vi "VecBuilder_8x1Fill.vi"(4 "R7":dbl, 5 "R0":dbl, 6 "R6":dbl, 7 "R1":dbl, 8 "R5":dbl, 9 "R4":dbl, 10 "R3":dbl, 11 "R2":dbl) -> (3 "output matrix":T1)   [LabVIEW 2019, in "Trajectory_Library.lvlib"]
doc: "Build a 8 x 1 Matrix (vector) from an array of input values.\n\nInputs:\n -- R0 -- Input value 1\n -- R1 -- Input value 2\n -- R2 -- Input value 3\n -- R3 -- Input value 4\n -- R4 -- Input value 5\n -- R5 -- Input value 6\n -- R6 -- Input value 7\n -- R7 -- Input value 8\n\nOutputs:\n -- Output Matrix -- Resulting 8 x 1 matrix (vector)"
uses:
  Trajectory_Library.lvlib
  <vilib>/Analysis/Matrix/Datatypes/RealMatrix.ctl
  <vilib>/Analysis/Matrix/NI_Matrix.lvlib
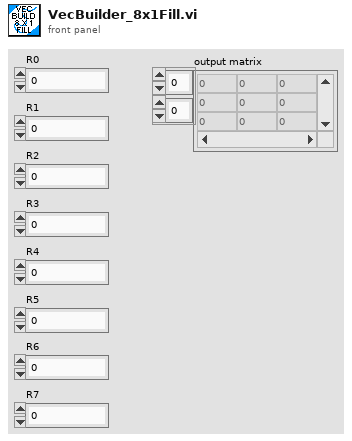
[diagram p1: front panel]
types:
  T1 = typedef "NI_Matrix.lvlib/RealMatrix.ctl" = dbl[][]
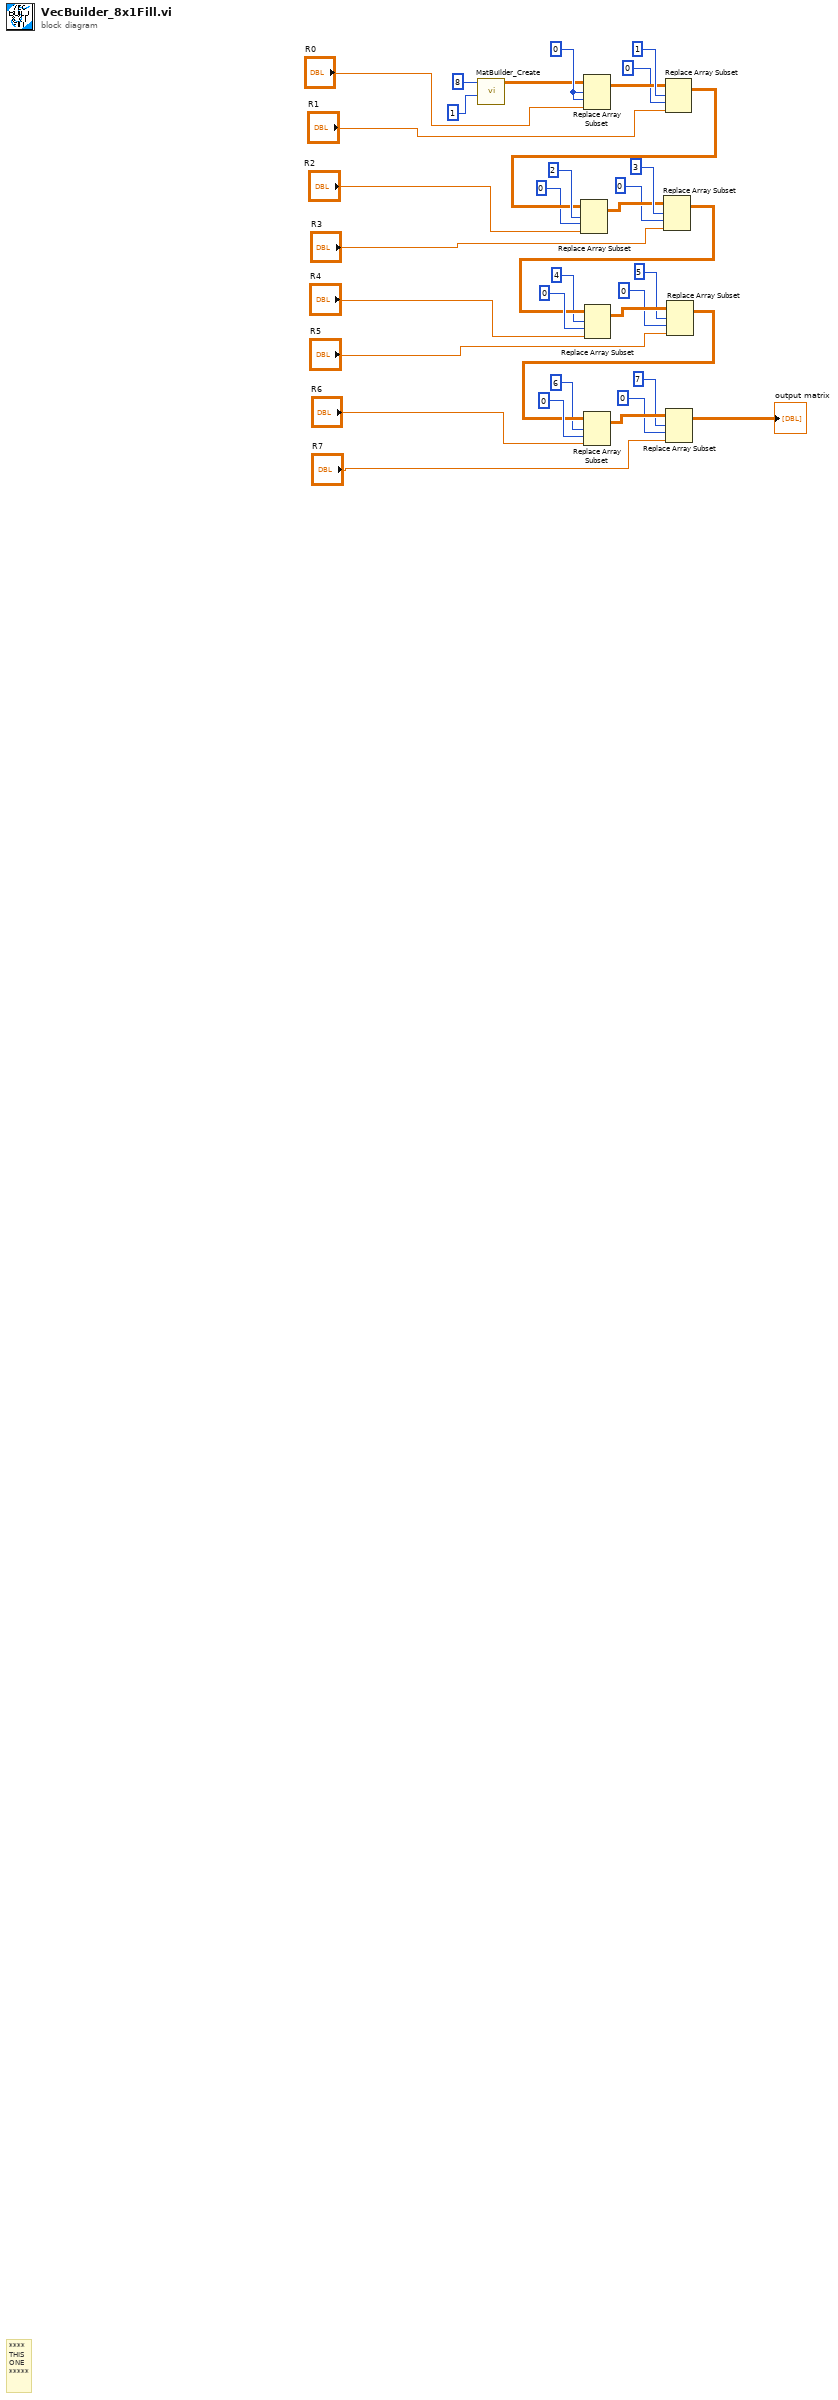
[diagram p0: block diagram]
diagram:
  w34 = 0 ("index (col)")
  # "****\nTHIS\nONE\n*****"
  n1 = call "MatBuilder_Create.vi"("Columns"=1, "Rows"=8) -> ("output matrix"=w22:T1)  [unwired: 9 in]
  n2 = Replace Array Subset(array=w22, new element="R0", index (row)=w34, index (col)=w34) -> (w32:T1)
  n3 = Replace Array Subset(array=w32, new element="R1", index (row)=1 ("index (col)"), index (col)=0 ("disabled index (col)")) -> (w26:T1)
  n4 = Replace Array Subset(array=w26, new element="R2", index (row)=2 ("index (col)"), index (col)=0 ("disabled index (col)")) -> (w25:T1)
  n5 = Replace Array Subset(array=w25, new element="R3", index (row)=3 ("index (col)"), index (col)=0 ("disabled index (col)")) -> (w15:T1)
  n6 = Replace Array Subset(array=w15, new element="R4", index (row)=4 ("index (col)"), index (col)=0 ("disabled index (col)")) -> (w21:T1)
  n7 = Replace Array Subset(array=w21, new element="R5", index (row)=5 ("index (col)"), index (col)=0 ("disabled index (col)")) -> (w14:T1)
  n8 = Replace Array Subset(array=w14, new element="R6", index (row)=6 ("index (col)"), index (col)=0 ("disabled index (col)")) -> (w18:T1)
  n9 = Replace Array Subset(array=w18, new element="R7", index (row)=7 ("index (col)"), index (col)=0 ("disabled index (col)")) -> (→"output matrix":T1)
